vi "Reentrant VI Execution.vi"() -> ()   [LabVIEW 2023]
doc: "This example program illustrates that each instance of a reentrant subvi has its own front panel and memory space. Only two instances are shown here, but the number of instances of a reentrant subvi is not limited in LabVIEW."
panel:
  in  "Open Instance 1":bool
  in  "Open Instance 0":bool
  in  "Stop":bool
  # "Overview: Demonstrates the functionality of Reentrant VIs.\nInstructions:\n1. Make sure no instances of Reentrant SubVI.vi are currently open.\n2. Run the VI.\n3. Click the Open Instance 0 button. The panel of the first reentrant subVI instance will open.\n4. Click the Open Instance 1 button. The panel of the second reentrant subVI instance will open.\n5. Click Stop on both reentrant subVI instance panels.\n6. Click Stop to stop this VI."
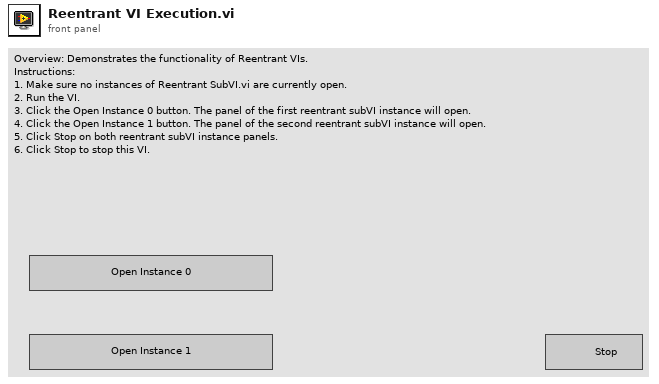
[diagram p1: front panel]
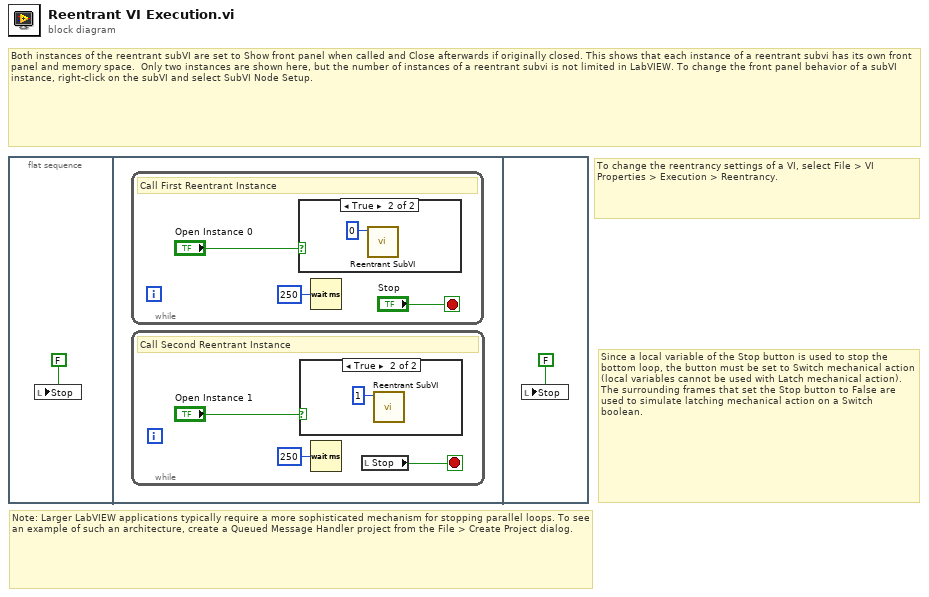
[diagram p0: block diagram]
diagram:
  # "To change the reentrancy settings of a VI, select File > VI Properties > Execution > Reentrancy."
  # "Since a local variable of the Stop button is used to stop the bottom loop, the button must be set to Switch mechanical action (local variables cannot be used with Latch mechanical action). The surrounding frames that set the Stop button to False are used to simulate latching mechanical action on a Switch boolean."
  # "Note: Larger LabVIEW applications typically require a more sophisticated mechanism for stopping parallel loops. To see an example of such an architecture, create a Queued Message Handler project from the File > Create Project dialog."
  # "Both instances of the reentrant subVI are set to Show front panel when called and Close afterwards if originally closed. This shows that each instance of a reentrant subvi has its own front panel and memory space.  Only two instances are shown here, but the number of instances of a reentrant subvi is not limited in LabVIEW. To change the front panel behavior of a subVI instance, right-click on the subVI and select SubVI Node Setup."
  n1 = flat-sequence {
    frame #0 {
      n2 = local write "Stop"(FALSE) -> ()
    }
    frame #1 {
      n3 = while {
        stop <- "Stop" stop-if-true
        # "Call First Reentrant Instance"
        n4 = case shown="True" "Open Instance 0" {
          frame False {
          }
          frame True {
            n5 = call "Reentrant SubVI.vi"("Instance"=0 ("Numeric Input")) -> ()  [unwired: 11 in]
          }
        }
        n6 = Wait (ms)(milliseconds to wait=u32 250 ("millisecond multiple")) -> ()  [unwired: 1 out]
      }
      n7 = while {
        stop <- w3 stop-if-true
        # "Call Second Reentrant Instance"
        n8 = case shown="True" "Open Instance 1" {
          frame False {
          }
          frame True {
            n9 = call "Reentrant SubVI.vi"("Instance"=1 ("Numeric Input")) -> ()  [unwired: 11 in]
          }
        }
        n10 = Wait (ms)(milliseconds to wait=u32 250 ("millisecond multiple")) -> ()  [unwired: 1 out]
        n11 = local read "Stop"() -> (w3:bool)
      }
    }
    frame #2 {
      n12 = local write "Stop"(FALSE) -> ()
    }
  }
